vi "log-fifo.vi"(8 "FIFO In":refnum<k21>="fpga-to-host2", 11 "input-data":fxp<+/-,25,6>[](array[numeric])=[0.0, 0.0, 0.0, 0.0, 0.0]) -> (3 "logging-timeout?":bool)   [LabVIEW 2015, in "FPGA-data-logging.lvlib"]
uses:
  <vilib>/rvi/DataTransferAndStorage/Container/Common/niFpgaContainerExecOnDevCompGetState.vi
  <vilib>/rvi/Emulation/niFpgaEmulationIsFPGAContextNoSignature.vi
  <vilib>/rvi/Emulation/niFpgaSctlEmulationGetInTimedLoop.vi
  <vilib>/rvi/errors/niFpgaSetErrorForExecOnDevCompSimple.vi
  <vilib>/rvi/eio/common/nirviEmuReportErrorAndStop.vi
  <vilib>/rvi/DataTransferAndStorage/Container/Common/niFpgaContainerGetUniqueNameForEmu.vi
  <vilib>/rvi/FIFO/Fifo_Resource/nirvififoEmulationSetSize.vi
  <vilib>/rvi/FIFO/Fifo_Resource/nirviFifoEmulationQueueMgr.vi
  <instcachedir>/0/nirviFifoEmulationQueueMgr_E5CAEC123FF24DC58D834DCA3CDAA9B5.lvgen/nirviFifoEmulationQueueMgr_E5CAEC123FF24DC58D834DCA3CDAA9B5_003.vi
  <vilib>/rvi/FIFO/Fifo_Resource/nirvififoEmulationDetermineInputValidOut.vi
  <vilib>/rvi/FIFO/Fifo_Resource/nirvififoEmulationCreateLock.vi
  <vilib>/rvi/Emulation/niFpgaProcessEmulError.vi
  <vilib>/rvi/FIFO/Fifo_Resource/nirvififoEmulationObtainLock.vi
  <vilib>/rvi/FIFO/Fifo_Resource/nirvififoEmulationReleaseLock.vi
  <vilib>/rvi/occurrence/nirviWaitOnOccurrenceBase.vi
  <vilib>/rvi/errors/nirviReportUnexpectedCaseInternalError.vi
  <vilib>/rvi/errors/nirviReportUnexpectedCaseInternalError (U32).vi
  <vilib>/Utility/error.llb/Clear Errors.vi
  <vilib>/rvi/interface/RandomDataEmulation/niFpgaRandomDataHandleErrors.vi
  <vilib>/rvi/DataTransferAndStorage/Container/XNode/niFpgaContainer.xnode
  <vilib>/rvi/FIFO/Fifo_Resource/niFpgaFifoEmulationRefIn.vi
  FPGA-data-logging.lvlib
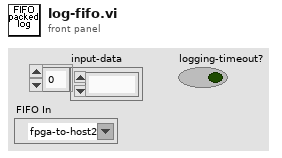
[diagram p1: front panel]
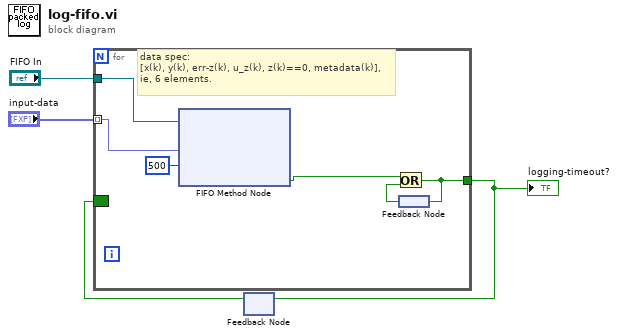
[diagram p0: block diagram]
diagram:
  n1 = feedback #1() -> (w2:bool)  [unwired: 1 in]
  n2 = for {
    tunnel: "input-data" -> [w10] mode=indexing
    tunnel: [w6] -> w4
    border: w2 -> [_]
    tunnel: "FIFO In" -> [w5]
    # "data spec:\n[x(k), y(k), err-z(k), u_z(k), z(k)==0, metadata(k)],\nie, 6 elements."
    n3 = xnode ("FIFO Method Node")("Element"=w10, "Timeout"=500, "FIFO In"=w5) -> ("Timed Out?"=w8:bool)  [unwired: 1 out]
    n4 = feedback #2() -> (w7:bool)
    n5 = Or(x=w8, y=w7) -> (x .or. y?=w6:bool)
    n6 = feedback-in #2(w6) -> ()
  }
  "logging-timeout?" <- w4
  n7 = feedback-in #1(w4) -> ()
